vi "append_array_example.vi"() -> ()   [LabVIEW 2019]
panel:
  out "Array":string[](array[string])
  out "concatenated string":string
  in  "Stop Button":bool
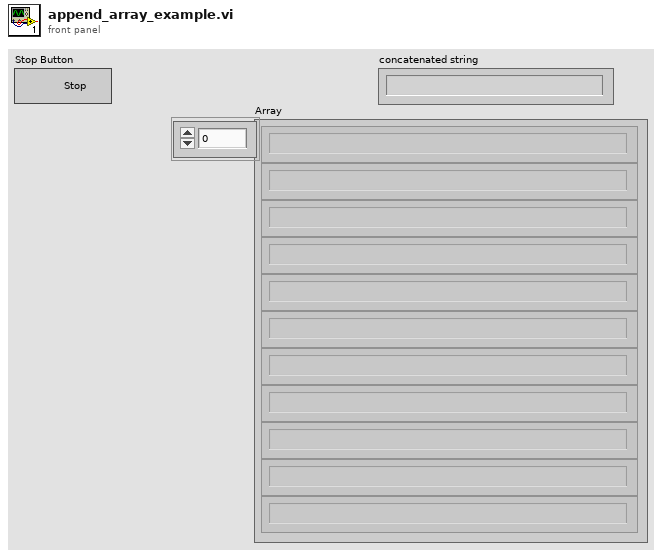
[diagram p1: front panel]
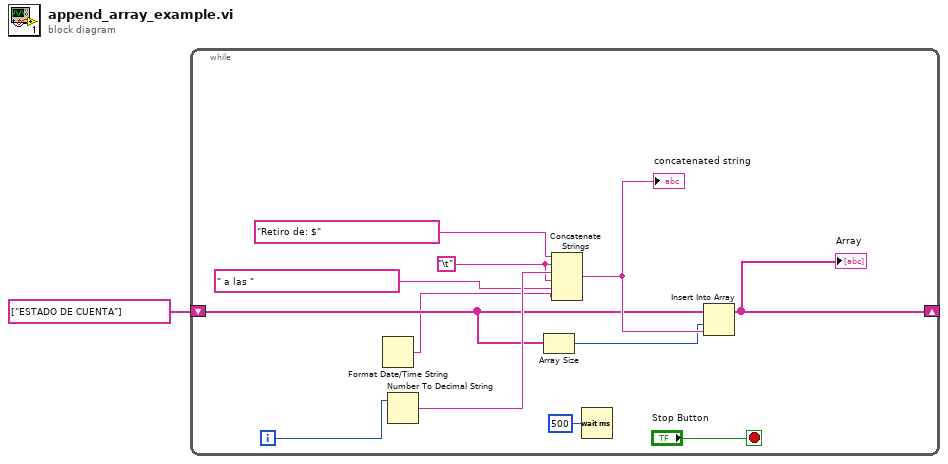
[diagram p0: block diagram]
diagram:
  n1 = while {
    shift-right: [w5] -> _
    shift-left: string[] ["ESTADO DE CUENTA"] -> [w7]
    i -> [w8]
    stop <- "Stop Button" stop-if-true
    w4 = "\t"
    n2 = Format Date/Time String() -> (date/time string=w3:string)  [unwired: 3 in]
    n3 = Number To Decimal String(number=w8) -> (decimal integer string=w10:string)  [unwired: 1 in]
    n4 = Array Size(array=w7) -> (size(s)=w6:i32)
    n5 = Concatenate Strings("Retiro de: $", w4, w10, w4, " a las ", w3) -> (w9:string)
    "concatenated string" <- w9
    n6 = Wait (ms)(milliseconds to wait=u32 500) -> ()  [unwired: 1 out]
    n7 = Insert Into Array(array=w7, index=w6, new element=w9) -> (w5:string[])
    "Array" <- w5
  }
